vi "createDAQmx.AI.vi"(8 "error in (no error)":errorcluster, 9 "DAQmx.AI.config":T1 {"input terminal configuration" items=["default"=-1, "RSE"=10083, "NRSE"=10078, "Differential"=10106, "Pseudodifferential"=12529]; "AI.Coupling" items=["AC"=10045, "DC"=10050, "GND"=10066]}, 10 "DAQ.config":T4={"Channels"="PXI1Slot2/ai0", "DAQ_Type"=enum."AI", "minimum value"=-5.0, "maximum value"=5.0, "DAQ_SamplingInfo"={"Fs"=0.0, "#s"=0}, "DAQ_SamplingMode"=enum."Continuous"} {"maximum value" format="%0.2f"; "minimum value" format="%0.2f"}, 11 "DAQmx.AI in":refnum<class "DAQmx.AI.lvclass">) -> (0 "error out":errorcluster, 3 "DAQmx.AI out":refnum<class "DAQmx.AI.lvclass">)   [LabVIEW 2020, in "DAQmx.AI.lvclass"]
uses:
  DAQmx.AI.lvclass
  C:/user/patrick/git/Multichannel-Lockin/src/SMOs/DAQmx/DAQmx.lvclass
  DAQ/Typedefs/DAQ_Config.ctl
  DAQ/Typedefs/PrivateEvents--DAQ.AI.Channels.ctl
  DAQ/Typedefs/DAQ_Type.ctl
  DAQ/Typedefs/DAQ_SamplingInfo.ctl
  DAQ/Typedefs/DAQ_SamplingMode.ctl
  Typedefs/DAQmx.AI_Config.ctl
  Typedefs/AI.Coupling-enum.ctl
  Typedefs/AI.Terminal-enum.ctl
  DAQmx.AI.lvclass/DAQmx.AI.ctl
  DAQmx/DAQmx.lvclass
  DAQ/DAQ.lvclass
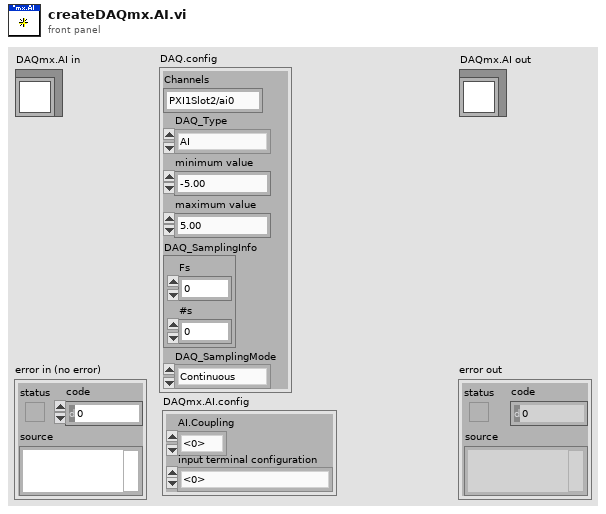
[diagram p1: front panel]
types:
  T1 = typedef "DAQmx.AI.lvclass/DAQmx.AI_Config.ctl" = cluster{"AI.Coupling":T2, "input terminal configuration ":T3}
  T2 = typedef "DAQmx.AI.lvclass/AI.Coupling-enum.ctl" = i32
  T3 = typedef "DAQmx.AI.lvclass/AI.Terminal-enum.ctl" = i32
  T4 = typedef "DAQ.lvclass/DAQ_Config.ctl" = cluster{"Channels":T5, "DAQ_Type":T6, "minimum value":dbl, "maximum value":dbl, "DAQ_SamplingInfo":T7, "DAQ_SamplingMode":T8}
  T5 = typedef "DAQ.lvclass/PrivateEvents--DAQ.AI.Channels.ctl" = string
  T6 = typedef "DAQ.lvclass/DAQ_Type.ctl" = enum16{"AI", "AO"}
  T7 = typedef "DAQ.lvclass/DAQ_SamplingInfo.ctl" = cluster{"Fs":dbl, "#s":i32}
  T8 = typedef "DAQ.lvclass/DAQ_SamplingMode.ctl" = enum16{"Continuous", "Finite"}
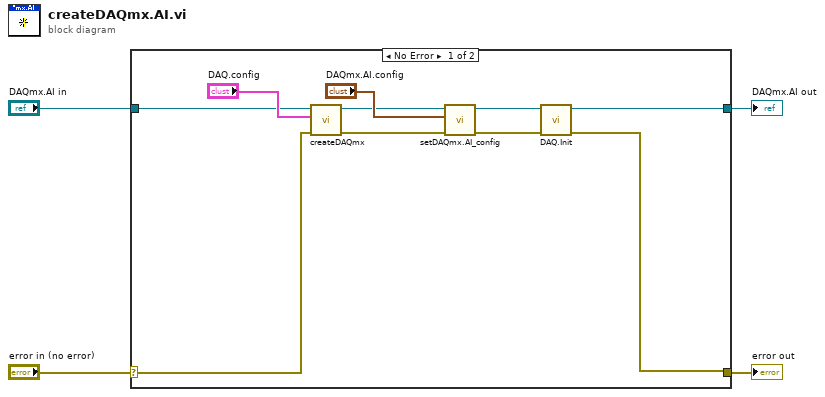
[diagram p0: block diagram]
diagram:
  n1 = case shown="No Error" "error in (no error)" {
    selector: "error in (no error)" -> [w12 w16]
    tunnel: [w11 w16] -> w3
    tunnel: [w10 w15] -> w1
    tunnel: "DAQmx.AI in" -> [w13 w15]
    frame No Error {
      n2 = call "createDAQmx.vi"("error in (no error)"=w12, "DAQ.Config"="DAQ.config", "DAQmx in"=w13) -> ("error out"=w5:errorcluster, "DAQmx out"=w8:refnum<class "DAQmx.AI.lvclass">)  [unwired: 7 in]
      n3 = call "setDAQmx.AI_config.vi"("error in (no error)"=w5, "DAQmx.AI_Config"="DAQmx.AI.config", "DAQmx.AI in"=w8) -> ("error out"=w6:errorcluster, "DAQmx.AI out"=w7:refnum<class "DAQmx.AI.lvclass">)  [unwired: 7 in]
      n4 = call-dynamic "DAQ.Init.vi"("error in (no error)"=w6, "DAQmx.AI in"=w7) -> ("error out"=w11:errorcluster, "DAQmx.AI out"=w10:refnum<class "DAQmx.AI.lvclass">)  [unwired: 8 in]
    }
    frame Error {
    }
  }
  "error out" <- w3
  "DAQmx.AI out" <- w1
